vi "SVFA Zoom FFT Spectrum (Mag-Phase) (N Ch).vi"(0 "scaled signals [EU]":waveform(dbl)[](array[waveform]), 3 "zoom settings":T2={"frequency range"={"start frequency"=1000.0, "stop frequency"=2000.0}, "window"=1, "number of lines"=400, "% overlap"=0.0} {"% overlap" min=0.0 format="%.2f"; "number of lines" min=2; "window" items=["None ", "Hanning", "Hamming", "Blackman-Harris", "Exact Blackman", "Blackman", "Flat Top", "4 Term B-Harris ", "7 Term B-Harris", "Low Sidelobe"]; "frequency range"."stop frequency" min=0.0 format="%.2f"; "frequency range"."start frequency" min=0.0 format="%.2f"}, 4 "view":T1={"dB On (T)"=TRUE, "unwrap phase (F)"=FALSE, "convert to degree (T)"=TRUE}, 5 "error in (no error)":errorcluster, 7 "averaging parameters":T9={"averaging mode"=enum."No averaging", "weighting mode"=enum."Exponential", "number of averages"=10, "linear mode"=enum."One shot"} {"number of averages" min=1 step=1}, 9 "restart averaging (F)":bool) -> (11 "averaging done":bool, 12 "new spectrum available":bool, 13 "averages completed":dbl, 14 "magnitudes [dB EU]":cluster{"f0":dbl, "df":dbl, "magnitude":dbl[]}[](array[cluster]) {"magnitude" format="%.2p"; "df" format="%.2p"; "f0" format="%.2p"}, 15 "magnitude unit labels":string[](array[string]), 16 "phases [degrees]":cluster{"f0":dbl, "df":dbl, "phase":dbl[]}[](array[cluster]) {"phase" format="%.2f"; "df" format="%.2f"; "f0" format="%.2f"}, 17 "phase unit labels":string[](array[string]), 18 "spectrum info":T3[](array[typedef]) {"x-axis units" items=["Time (s)"=0, "Frequency-CB (Hz)"=1, "Frequency-CPB (Hz)"=1248, "Frequency-Arbitrary (Hz)"=2357, "Quefrency (s)"=2, "Revolutions (rev)"=3, "Order"=4, "Speed (RPM)"=11, "Speed (rad/s)"=21, "Index"=65535]; "weighting filter" items=["Linear", "A-weighting", "B-weighting", "C-weighting", "ITU-R 468-4", "Dolby", "CCITT", "C-message", "Wb", "Wc", "Wd", "We", "Wf", "Wh", "Wj", "Wk", "Wm", "AES17 20 kHz lowpass", "AES17 40 kHz lowpass", "AES17 20 kHz highpass", "AES17 40 kHz highpass"]; "dB reference [EU]" format="%.2f"; "engineering units" items=["custom..."=0, "V"=1, "A"=21, "C"=30, "pC"=31, "s"=32, "-"=29, "Pa"=2, "N"=20, "g"=3, "m/s^2"=4, "m/s"=5, "m"=6, "mm/s"=12, "mm"=13, "micron/s"=14, "micron"=15, "in/s^2"=7, "in/s"=8, "in"=9, "mil/s"=10, "mil"=11, "rad/s^2"=16, "rad/s"=17, "rad"=18, "deg/s^2"=26, "deg/s"=27, "deg"=28, "RPM"=22, "cycle/s^2"=23, "Hz"=24, "cycle"=25, "strain"=19]; "spectral info"."window" items=["None "=0, "Hanning"=1, "Hamming"=2, "Blackman-Harris"=3, "Exact Blackman"=4, "Blackman"=5, "Flat Top"=6, "4 Term B-Harris "=7, "7 Term B-Harris"=8, "Low Sidelobe"=9, "Force - Exponential"=10, "Gaussian"=62]}, 19 "error out":errorcluster)   [LabVIEW 2017]
doc: "Computes the zoom FFT spectrum of <B>scaled signal [EU]</B> and <B>zoom settings</B>. Zoom FFT results are returned in magnitude and phase. Data accumulates each time this VI is called. However, it returns a new spectrum only when sufficient data accumulates. Indicators and subsequent processing should only be called when <B>new spectrum available</B> is TRUE. Wire data to the <B>scaled signal [EU]</B> input to determine the polymorphic instance to use or manually select the instance."
uses:
  <vilib>/addons/_NISVFA/_Shared subVIs/Controls/svc_Spectrum Info.ctl
  <vilib>/addons/_NISVFA/_Shared subVIs/Controls/svc_X-Axis Units.ctl
  <vilib>/addons/_NISVFA/_Shared subVIs/Controls/svc_Spectrum Type.ctl
  <vilib>/addons/_NISVFA/_Shared subVIs/Controls/svc_Engineering Units Text Ring.ctl
  <vilib>/addons/_NISVFA/_Shared subVIs/Controls/svc_Weighting Filter Text Ring.ctl
  <vilib>/addons/_NISVFA/_Shared subVIs/Controls/svc_Complimentary Spectrum Units.ctl
  <vilib>/addons/_NISVFA/_Shared subVIs/Spectrum Info/svfa_Build Spectrum Info.vi
  <vilib>/addons/_NISVFA/_Shared subVIs/Spectrum Averaging/svfa_Reset Averaging State Info.vi
  <vilib>/addons/_NISVFA/_Shared subVIs/Spectrum Averaging/svfa_Average Array with Avg Checks (complex) No State.vi
  <vilib>/addons/_NISVFA/_Shared subVIs/Common/svc_Complex to Mag2 Array.vi
  <vilib>/addons/_NISVFA/_Shared subVIs/Spectrum Averaging/svfa_Average Array with Avg Checks (real) No State.vi
  <vilib>/addons/_NISVFA/_Shared subVIs/Common/svc_Get SV Channel Info.vi
  <vilib>/addons/_NISVFA/_Shared subVIs/Common/svc_Spectrum Units.vi
  <vilib>/addons/_NISVFA/_Shared subVIs/Spectrum Averaging/svfa_Average Array (complex) No State.vi
  <vilib>/addons/_NISVFA/_Shared subVIs/Spectrum Averaging/svfa_Average Array (real) No State.vi
  <vilib>/addons/_NISVFA/_Shared subVIs/Spectrum Averaging/svfa_No Average Array (complex).vi
  <vilib>/addons/_NISVFA/_Shared subVIs/Spectrum Averaging/svfa_Average Array (complex).vi
  <vilib>/addons/_NISVFA/_Shared subVIs/Spectrum Averaging/svfa_No Average Array (real).vi
  <vilib>/addons/_NISVFA/_Shared subVIs/Spectrum Averaging/svfa_Average Array (real).vi
  <vilib>/addons/_NISVFA/_Shared subVIs/Spectrum Averaging/svfa_Peak Hold Array.vi
  <vilib>/addons/_NISVFA/_Shared subVIs/Common/svc_Get Weighting Enum and Labels.vi
  <vilib>/addons/_NISVFA/_Shared subVIs/Common/svc_Unit Label Lexical Class.vi
  <vilib>/addons/_NISVFA/_Shared subVIs/Common/svc_Engineering Units to Unit Label.vi
  <vilib>/addons/_NISVFA/_Shared subVIs/Common/svc_Format Value (DBL).vi
  <vilib>/addons/_NISVFA/_Shared subVIs/Common/svc_Channel Info to Spectrum Info.vi
  <vilib>/addons/_NISVFA/_Shared subVIs/Common/svc_Unit Label to Engineering Units.vi
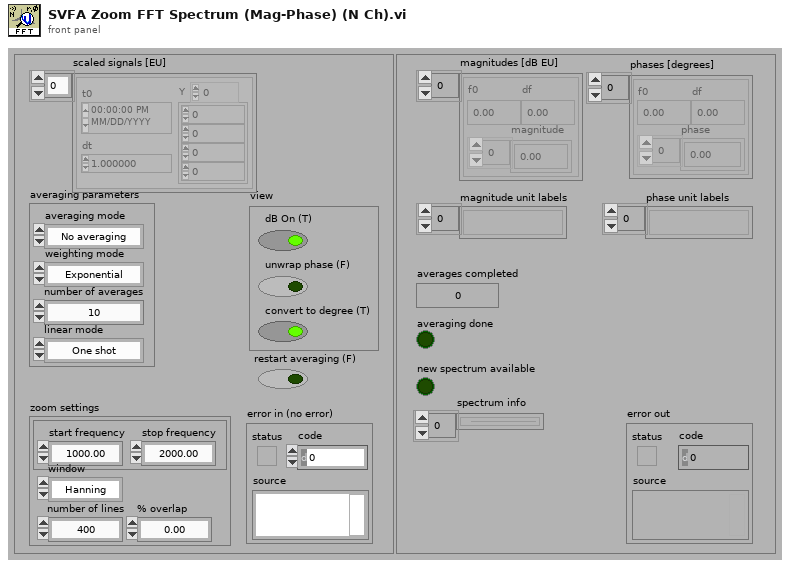
[diagram p1: front panel]
types:
  T1 = cluster{"dB On (T)":bool, "unwrap phase (F)":bool, "convert to degree (T)":bool}
  T2 = cluster{"frequency range":cluster{"start frequency":dbl, "stop frequency":dbl}, "window":u16, "number of lines":i32, "% overlap":dbl}
  T3 = typedef "svc_Spectrum Info.ctl" = cluster{"channel name":string, "description":string, "x-axis units":T4, "spectral info":cluster{"spectrum type":T5, "linear/dB":enum16{"linear", "dB"}, "window":u16, "window size":i32, "FFT size":i32}, "engineering units":T6, "custom label":string, "dB reference [EU]":dbl, "peak units":enum16{"rms", "peak", "peak-peak"}, "weighting filter":T7, "spectral density?":bool, "unit label":string, "spectrum skewed?":bool, "complimentary spectrum units":T8}
  T4 = typedef "svc_X-Axis Units.ctl" = u16
  T5 = typedef "svc_Spectrum Type.ctl" = enum16{"FFT Spectrum [complex]", "Amplitude [Magnitude]", "Power [Magnitude^2]", "Cross Spectrum [complex]", "Frequency Response [Complex]"}
  T6 = typedef "svc_Engineering Units Text Ring.ctl" = u16
  T7 = typedef "svc_Weighting Filter Text Ring.ctl" = u16
  T8 = typedef "svc_Complimentary Spectrum Units.ctl" = enum16{"none", "radians", "degrees", "cycles", "imaginary"}
  T9 = cluster{"averaging mode":enum16{"No averaging", "Vector averaging", "RMS averaging", "Peak hold"}, "weighting mode":enum16{"Linear", "Exponential"}, "number of averages":u32, "linear mode":enum16{"One shot", "Auto restart"}}
  T10 = enum16{"Restart processing", "Continue processing", "Skip processing"}
  T11 = enum16{"No averaging", "Vector averaging", "RMS averaging", "Peak hold"}
  T12 = cluster{"f0":dbl, "df":dbl, "complex FFT":cdb[]}[]
  T13 = cluster{"zoom settings":cluster{"center frequency":dbl, "zoom":i32, "trim":dbl}, "FFT settings":cluster{"window":enum16{"None ", "Hanning", "Hamming", "Blackman-Harris", "Exact Blackman", "Blackman", "Flat Top", "4 Term B-Harris ", "7 Term B-Harris", "Low Sidelobe"}, "window size":i32, "FFT size":i32, "%overlap":dbl}}
  T14 = cluster{"complex FFT":cdb[], "real FFT":dbl[], "f0":dbl, "df":dbl, "averages completed":dbl, "averaging parameters":cluster{"averaging mode":enum16{"No averaging", "Vector averaging", "RMS averaging", "Peak hold"}, "weighting mode":enum16{"Linear", "Exponential"}, "number of averages":u32, "linear mode":enum16{"One shot", "Auto restart"}}}[]
  T15 = cluster{"complex FFT":cdb[], "real FFT":dbl[], "f0":dbl, "df":dbl, "averages completed":dbl, "averaging parameters":cluster{"averaging mode":enum16{"No averaging", "Vector averaging", "RMS averaging", "Peak hold"}, "weighting mode":enum16{"Linear", "Exponential"}, "number of averages":u32, "linear mode":enum16{"One shot", "Auto restart"}}}
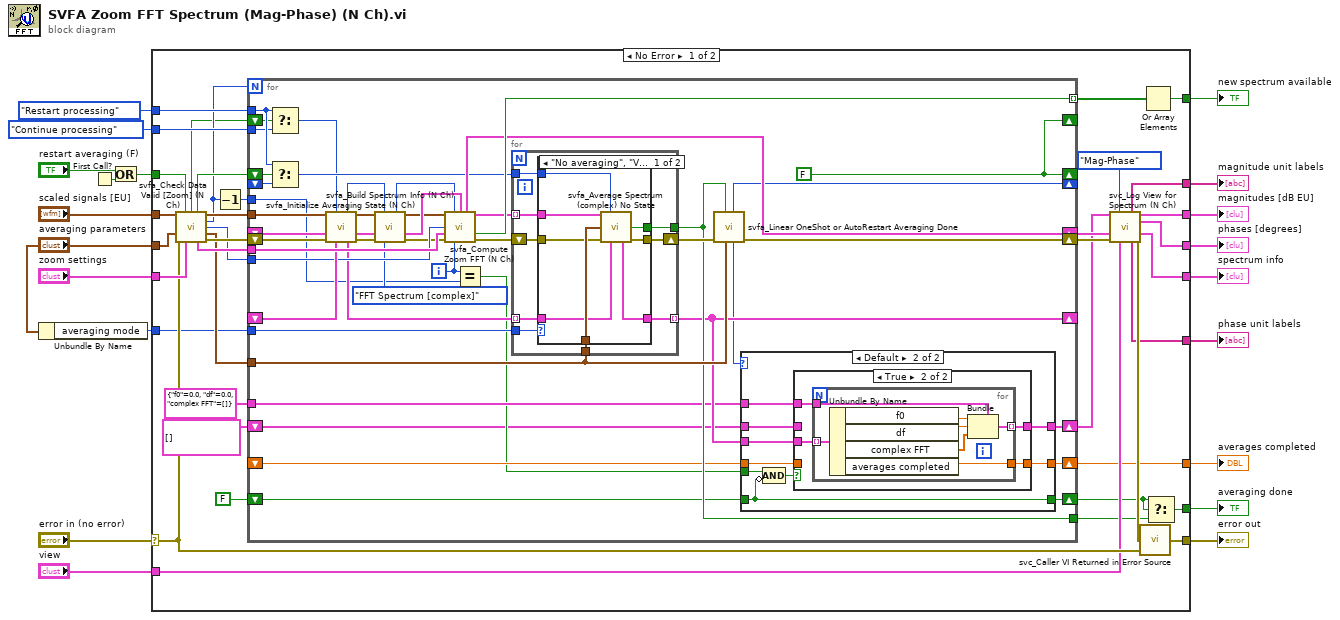
[diagram p0: block diagram]
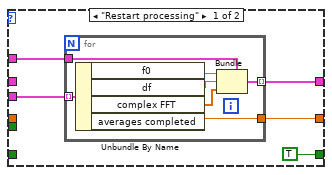
[diagram p2: hidden frame]
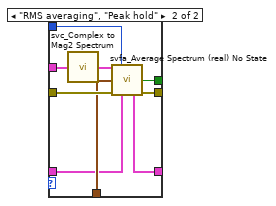
[diagram p4: hidden frame]
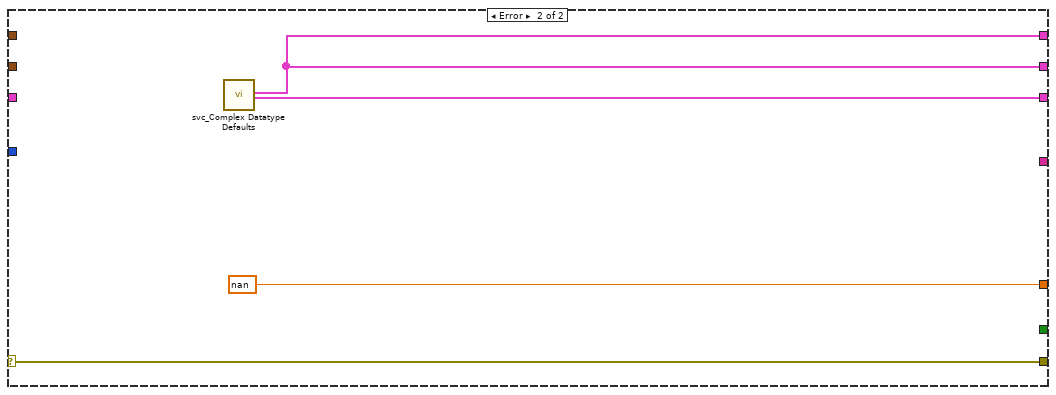
[diagram p5: hidden frame]
diagram:
  n1 = Unbundle By Name("averaging parameters") -> ("averaging mode"=w1:T11)
  n2 = First Call?() -> (First Call?: T/F=w7:bool)
  n3 = Or(x="restart averaging (F)", y=w7) -> (x .or. y?=w5:bool)
  n4 = case shown="No Error" "error in (no error)" {
    selector: "error in (no error)" -> [w47 w167]
    tunnel: w5 -> [w35 _]
    tunnel: [w22 nan ("Averaged So-far")] -> w20
    tunnel: [w36 _] -> w19
    tunnel: [w40 w167] -> w18
    tunnel: "averaging parameters" -> [w46 _]
    tunnel: "zoom settings" -> [w48 _]
    tunnel: "scaled signals [EU]" -> [w49 _]
    tunnel: [w39 w164] -> w8
    tunnel: [w38 _] -> w14
    tunnel: [w43 _] -> w13
    tunnel: [w41 w165] -> w12
    tunnel: [w42 w165] -> w11
    tunnel: [w29 _] -> w10
    tunnel: "view" -> [w45 _]
    tunnel: T10."Restart processing" ("processing control in") -> [w34 _]
    tunnel: T10."Continue processing" ("processing control in") -> [w33 _]
    tunnel: w1 -> [w27 _]
    frame No Error {
      n5 = call <vilib>:"svfa_Check Data Valid [Zoom] (N Ch).vi"("scaled signals [EU]"=w49, "restart averaging (F)"=w35, "averaging parameters"=w46, "error in (no error)"=w47, "zoom settings"=w48) -> ("reset processing"=w31:bool, "restart averaging"=w50:bool, "dup scaled signals"=w56:waveform(dbl)[], "iterations"=w32:i32, "maximum block size"=w37:i32, "dup averaging parameters"=w53:T9, "zoom FFT settings"=w54:T13, "error out"=w55:errorcluster)  [unwired: 3 in]
      n6 = Decrement(x=w32) -> (x-1=w30:i32)
      n7 = for {
        N: w32 -> [_]
        shift-left: _ -> [w98]
        shift-right: [w67] -> _
        tunnel: [w99] -> w44 mode=indexing
        tunnel: w54 -> [w101]
        tunnel: w56 -> [w102]
        tunnel: [w71] -> w28
        tunnel: w53 -> [w95]
        shift-right: [w97] -> w51
        shift-left: _ -> [w96]
        shift-right: [w59] -> _
        shift-left: _ -> [w94]
        tunnel: w34 -> [w91]
        tunnel: w37 -> [w92]
        shift-right: [w64] -> _
        shift-left: w50 -> [w93]
        tunnel: w33 -> [w90]
        tunnel: w30 -> [w72]
        shift-right: [w103] -> w52
        shift-left: w55 -> [w100]
        shift-right: [w64] -> _
        shift-left: w31 -> [w74]
        tunnel: w27 -> [w70]
        shift-right: [w65] -> w21
        shift-left: T12 [] -> [w60]
        shift-right: [w69] -> w23
        shift-left: FALSE ("restart averaging") -> [w61]
        shift-right: [w68] -> w22
        shift-left: _ -> [w63]
        tunnel: cluster{"f0":dbl, "df":dbl, "complex FFT":cdb[]} {"f0"=0.0, "df"=0.0, "complex FFT"=[]} -> [w66]
        i -> [w73]
        w64 = FALSE ("restart averaging")
        n8 = Select(t=w91, s=w74, f=w90) -> (s? t:f=w75:T10)
        n9 = Select(t=w91, s=w93, f=w94) -> (s? t:f=w76:T10)
        n10 = call <vilib>:"svfa_Initialize Averaging State (N Ch).vi"("Windowed Waveform(s)"=w102, "processing control in"=w75, "spectra info in"=w96, "error in (no error)"=w100, "state info"=w98) -> ("processing control out"=w81:T10, "Windowed Waveform(s)"=w83:waveform(dbl)[], "spectra info out"=w82:T3[], "state info"=w79:T14, "error out"=w84:errorcluster)  [unwired: 6 in]
        n11 = call <vilib>:"svfa_Build Spectrum Info (N Ch).vi"("scaled signal(s)"=w83, "processing control in"=w81, "spectra info in"=w82, "error in (no error)"=w84, "spectrum type"=svc_Spectrum_Type."FFT Spectrum [complex]") -> ("dup processing control"=w78:T10, "dup scaled signals"=w80:waveform(dbl)[], "spectra info out"=w88:T3[], "error out"=w77:errorcluster)  [unwired: 7 in]
        n12 = call <vilib>:"svfa_Compute Zoom FFT (N Ch).vi"("scaled signals [EU]"=w80, "processing control"=w78, "spectra info in"=w88, "maximum block size"=w92, "zoom FFT settings"=w101, "error in (no error)"=w77, "iteration"=w73) -> ("spectra info out"=w97:T3[], "FFT spectra"=w86:cluster{"f0":dbl, "df":dbl, "spectrum":cdb[]}[], "spectrum ready"=w99:bool, "error out"=w85:errorcluster)  [unwired: 4 in, 1 out]
        n13 = Equal?(x=w73, y=w72) -> (x = y?=w62:bool)
        n14 = for {
          tunnel: w95 -> [w146]
          tunnel: w70 -> [w145]
          tunnel: [w143] -> w71
          tunnel: [w142] -> w67 mode=indexing
          tunnel: w86 -> [w141] mode=indexing
          tunnel: w76 -> [w139]
          tunnel: w79 -> [w138] mode=indexing
          shift-right: [w144] -> w89
          shift-left: w85 -> [w140]
          n15 = case shown="\"No averaging\", \"Vector averaging\"" w145 {
            tunnel: w146 -> [w153 w161]
            tunnel: [w151 w157] -> w144
            tunnel: [w150 w162] -> w143
            tunnel: w141 -> [w154 w158]
            tunnel: w140 -> [w152 w163]
            tunnel: w139 -> [w149 w159]
            tunnel: [w148 w155] -> w142
            tunnel: w138 -> [w147 w156]
            frame "No averaging", "Vector averaging" {
              n16 = call <vilib>:"svfa_Average Spectrum (complex) No State.vi"("spectrum"=w154, "processing control"=w149, "averaging parameters"=w153, "error in (no error)"=w152, "averaging state info in"=w147) -> ("averaging done"=w150:bool, "averaging state info out"=w148:T15, "error out"=w151:errorcluster)  [unwired: 5 in, 3 out]
            }
            frame "RMS averaging", "Peak hold" {
              n17 = call <vilib>:"svc_Complex to Mag2 Spectrum.vi"("complex spectrum"=w158) -> ("power spectrum"=w160:cluster{"f0":dbl, "df":dbl, "spectrum":dbl[]})  [unwired: 4 in]
              n18 = call <vilib>:"svfa_Average Spectrum (real) No State.vi"("spectrum"=w160, "processing control"=w159, "averaging parameters"=w161, "error in (no error)"=w163, "averaging state info in"=w156) -> ("averaging done"=w162:bool, "averaging state info out"=w155:T15, "error out"=w157:errorcluster)  [unwired: 5 in, 3 out]
            }
          }
        }
        n19 = call <vilib>:"svfa_Linear OneShot or AutoRestart Averaging Done.vi"("averaging parameters"=w95, "averaging done"=w71, "error in (no error)"=w89) -> ("error out"=w103:errorcluster, "processing control"=w59:T10)  [unwired: 7 in]
        n20 = case shown="Default" w59 {
          tunnel: w67 -> [w108 w124]
          tunnel: [TRUE ("restart averaging") w119] -> w69
          tunnel: [w106 w123] -> w65
          tunnel: w61 -> [_ w119]
          tunnel: w62 -> [_ w122]
          tunnel: w66 -> [w105 w121]
          tunnel: [w104 w118] -> w68
          tunnel: w63 -> [_ w117]
          tunnel: w60 -> [_ w116]
          frame "Restart processing" {
            n21 = for {
              tunnel: w108 -> [w112] mode=indexing
              tunnel: [w111] -> w106 mode=indexing
              tunnel: w105 -> [w110]
              tunnel: [w109] -> w104
              n22 = Unbundle By Name(w112) -> ("f0"=w115:dbl, "df"=w114:dbl, "complex FFT"=w113:cdb[], "averages completed"=w109:dbl)
              n23 = Bundle(cluster=w110, "f0"=w115, "df"=w114, "complex FFT"=w113) -> (w111:cluster{"f0":dbl, "df":dbl, "complex FFT":cdb[]})
            }
          }
          frame Default {
            n24 = Compound Arithmetic op=AND(w122, invert w119) -> (w120:bool)
            n25 = case shown="True" w120 {
              tunnel: w124 -> [_ w130]
              tunnel: [w125 w129] -> w123
              tunnel: w121 -> [_ w128]
              tunnel: [w126 w127] -> w118
              tunnel: w117 -> [w126 _]
              tunnel: w116 -> [w125 _]
              frame False {
              }
              frame True {
                n26 = for {
                  tunnel: w130 -> [w134] mode=indexing
                  tunnel: [w133] -> w129 mode=indexing
                  tunnel: w128 -> [w132]
                  tunnel: [w131] -> w127
                  n27 = Unbundle By Name(w134) -> ("f0"=w137:dbl, "df"=w136:dbl, "complex FFT"=w135:cdb[], "averages completed"=w131:dbl)
                  n28 = Bundle(cluster=w132, "f0"=w137, "df"=w136, "complex FFT"=w135) -> (w133:cluster{"f0":dbl, "df":dbl, "complex FFT":cdb[]})
                }
              }
            }
          }
        }
      }
      n29 = call <vilib>:"svc_Log View for Spectrum (N Ch).vi"("complex spectra"=w21, "View"=enum16{"Mag-Phase", "Real-Imaginary"}."Mag-Phase", "spectra info in"=w51, "error in (no error)"=w52, "view"=w45) -> ("unit label [mag or real]"=w43:string[], "magnitude or real"=w42:cluster{"f0":dbl, "df":dbl, "magnitude":dbl[]}[], "phase or imaginary"=w41:cluster{"f0":dbl, "df":dbl, "magnitude":dbl[]}[], "spectra info out"=w39:T3[], "unit label [phase or imag]"=w38:string[], "error out"=w58:errorcluster)  [unwired: 5 in]
      n30 = call <vilib>:"svc_Caller VI Returned in Error Source.vi"("warning input to caller"=w47, "error in (no error)"=w58) -> ("error out"=w40:errorcluster)  [unwired: 3 in]
      n31 = Or Array Elements(Boolean array=w44) -> (logical OR=w36:bool)
      n32 = Select(t=w23, s=w23, f=w28) -> (s? t:f=w29:bool)
    }
    frame Error {
      n33 = call <vilib>:"svc_Complex Datatype Defaults.vi"() -> ("empty array of spectra"=w165:cluster{"f0":dbl, "df":dbl, "magnitude":dbl[]}[], "empty array of spectrum info"=w164:T3[])  [unwired: 11 in, 7 out]
    }
  }
  "averages completed" <- w20
  "new spectrum available" <- w19
  "error out" <- w18
  "spectrum info" <- w8
  "magnitude unit labels" <- w13
  "phase unit labels" <- w14
  "magnitudes [dB EU]" <- w11
  "phases [degrees]" <- w12
  "averaging done" <- w10
